vi "Msg.Event.Destroy.vi"(8 "Error (in)":errorcluster, 11 "Msg.Event.Ref":T1) -> (0 "Error (out)":errorcluster)   [LabVIEW 2023, in "MessagingModule.lvlib"]
doc: "Used to destroy a user event."
uses:
  Msg.Event.Ref.ctl
  Msg.Data.ctl
  MessagingModule.lvlib
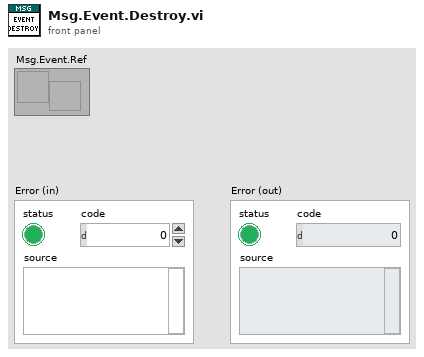
[diagram p1: front panel]
types:
  T1 = typedef "MessagingModule.lvlib/Msg.Event.Ref.ctl" = refnum<user-event>
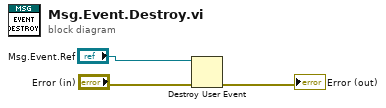
[diagram p0: block diagram]
diagram:
  n1 = Destroy User Event(user event="Msg.Event.Ref", error in="Error (in)") -> (error out=→"Error (out)":errorcluster)
